vi "Configure Shunt.vi"(8 "error in (no error)":errorcluster, 10 "Shunt (Internal)":u16(ring) items=["Internal", "External"], 11 "VISA resource name":refnum<visa-resource-name>) -> (0 "error out":errorcluster, 3 "VISA resource name out":refnum<visa-resource-name>)   [LabVIEW 2015, in "Voltech PM1000+.lvlib"]
doc: "Configures internal or external shunt for current shunt. It also indicates the shunt settings.\n\nThe internal shunt of the PM1000+ is suitable for measurements in the range 20mA to 20A rms and this may be extended by the use of suitable current transducers from uA to MA.\n\nSome current transducers (including simple resistive shunts) produce a voltage that is proportional to current. External Shunt Inputs are provided on the PM1000+ for use with current transducers that provide a voltage output.\n\nBecause the 0V is common to both the internal and external shunts, only one\ntype may be connected at any time."
uses:
  <instrlib>/Voltech PM1000+/Voltech PM1000+.lvlib
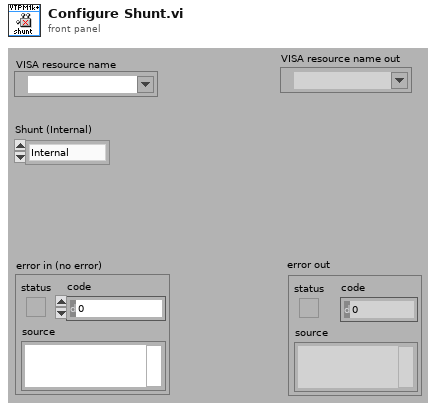
[diagram p1: front panel]
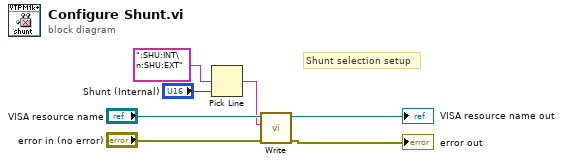
[diagram p0: block diagram]
diagram:
  # "Shunt selection setup"
  n1 = Pick Line(multi-line string=":SHU:INT\n:SHU:EXT", line index="Shunt (Internal)") -> (output string=w3:string)  [unwired: 1 in]
  n2 = call <instrlib>:"Write.vi"("error in (no error)"="error in (no error)", "Write Buffer"=w3, "VISA resource name"="VISA resource name") -> ("error out"=→"error out":errorcluster, "VISA resource name out"=→"VISA resource name out":refnum<visa-resource-name>)  [unwired: 7 in]
